vi "Read Result file path.vi"(8 "error in (no error)":errorcluster, 11 "HC-ScanParser in":refnum<class "HC-ScanParser.lvclass">) -> (0 "error out":errorcluster, 2 "Result file path":path, 3 "HC-ScanParser out":refnum<class "HC-ScanParser.lvclass">)   [LabVIEW 2013, in "HardwareCharacterization.lvlib" / "HC-ScanParser.lvclass"]
uses:
  HC-ScanParser.lvclass
  HC-ScanParser.lvclass/HC-ScanParser.ctl
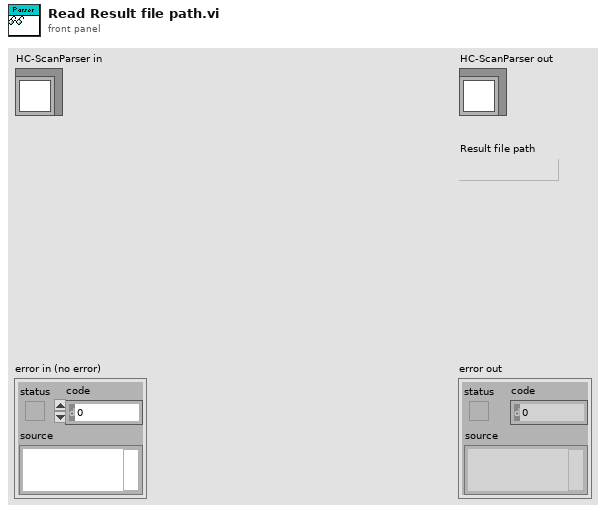
[diagram p1: front panel]
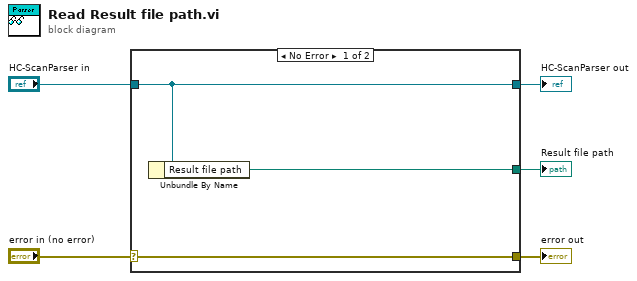
[diagram p0: block diagram]
diagram:
  n1 = case shown="No Error" "error in (no error)" {
    selector: "error in (no error)" -> [w8 w9]
    tunnel: [w8 w9] -> w4
    tunnel: [w7 w10] -> w2
    tunnel: "HC-ScanParser in" -> [w7 w10]
    tunnel: [w6 _] -> w1
    frame No Error {
      n2 = Unbundle By Name(w7) -> ("Result file path"=w6:path)
    }
    frame Error {
    }
  }
  "error out" <- w4
  "HC-ScanParser out" <- w2
  "Result file path" <- w1
